vi "2ndOrderTF_v1.vi"(7 "Enable?":bool, 9 "Denominator":fxp<+/-,18,3>[](array[numeric])=[0.0, 0.0], 10 "Numerator":fxp<+/-,18,3>[](array[numeric])=[0.0, 0.0, 0.0], 11 "Input":fxp<+/-,25,4>) -> (3 "Output":fxp<+/-,25,4> format="%.29g")   [LabVIEW 2017, in "FPGA Controllers.lvlib"]
doc: "2nd order TF. Use this for implementing a notch filter.\n\nImplements, u(k) = a0*e(k-2) + a1*e(k-1) + a2*e(k) - b0*u(k-2) - b1*u(k-1)\n\nSet parameters, Num = a0, a1, a2 and Den = b0, b1"
uses:
  FPGA Controllers.lvlib
  <vilib>/rvi/FXPMathLib/basic elements/FxpDiscreteDelay/XNode/nifxpmath_DiscreteDelay.xnode
  <vilib>/Platform/TimedLoop/XDataNode/XDataNode.xnode
  <vilib>/Platform/TimedLoop/XDataNode/nitl_modes.ctl
  <vilib>/Platform/TimedLoop/XDataNode/XDNodeRunTimeDep.lvlib
  <vilib>/Platform/TimedLoop/XDataNode/wakeup.ctl
  <vilib>/Platform/TimedLoop/XDataNode/timing_clust.ctl
  <vilib>/rvi/FXPMathLib/FxpMul/XNode/nifxpmath_Multiplier.xnode
  <vilib>/rvi/FXPMathLib/sim/FxpSim.dll
  <vilib>/rvi/FXPMathLib/FxpAdd/XNode/nifxpmath_Add.xnode
  <vilib>/rvi/FXPMathLib/FxpSub/XNode/nifxpmath_Sub.xnode
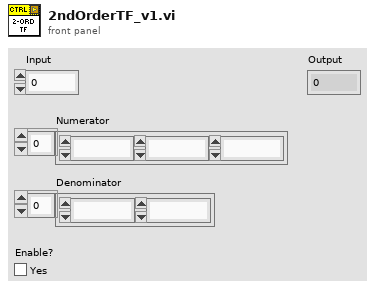
[diagram p1: front panel]
types:
  T1 = typedef "XDNodeRunTimeDep.lvlib/timing_clust.ctl" = cluster{"Expected End [f-1]":u64, "Actual End [f-1]":u64, "Finished Late? [f-1]":bool, "Expected End [i-1]":u64, "Actual End [i-1]":u64, "Finished Late? [i-1]":bool, "Expected Start [i]":u64, "Actual Start [i]":u64, "Expected Start [f]":u64, "Actual Start [f]":u64, "Source Name":string, "Structure Name":string, "Period":i64, "Deadline":i64, "Offset":i64, "Start":i64, "Priority":i32, "Timeout":i32, "Mode":T2, "Wakeup Reason":T3, "Error":errorcluster, "Source Type":string, "Secondary Source Type":string, "Global End Time":u64, "Global Start Time":u64, "Frame Duration":u64, "Iteration Duration":u64, "Assigned CPU":i32, "I/O Scan Engine Mode":u32}
  T2 = typedef "XDNodeRunTimeDep.lvlib/nitl_modes.ctl" = enum32{"No Change", "Process missed periods, maintain original phase", "Discard missed periods, maintain original phase", "Process missed periods, ignore original phase", "Discard missed periods, ignore original phase"}
  T3 = typedef "XDNodeRunTimeDep.lvlib/wakeup.ctl" = enum32{"Normal", "Aborted", "Asynchronous wakeup", "Timing source error", "Timed loop error", "Timeout"}
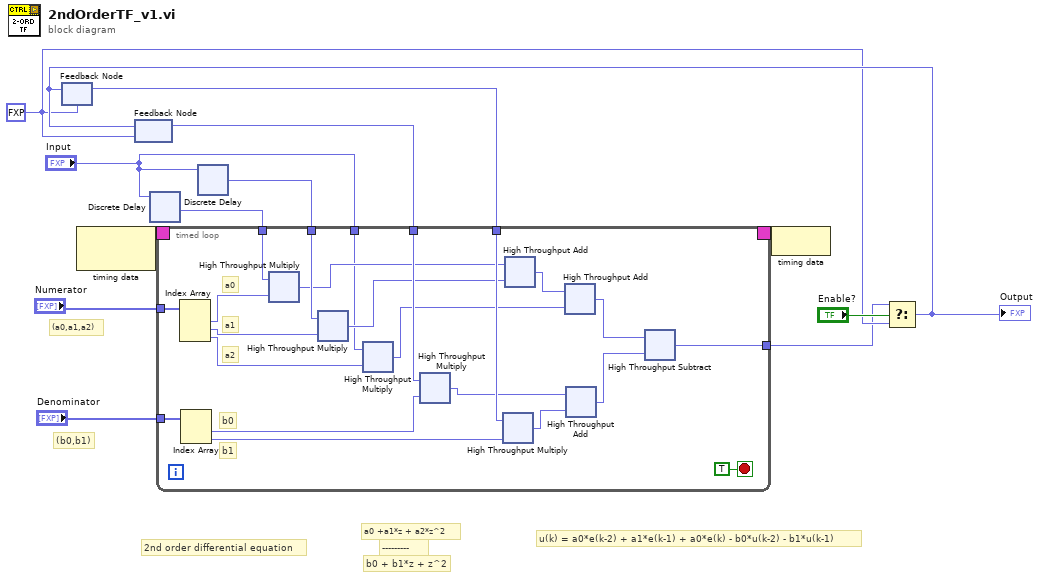
[diagram p0: block diagram]
diagram:
  w4 = fxp<+/-,25,4> 0.0 ("Input")
  # "2nd order differential equation"
  # "u(k) = a0*e(k-2) + a1*e(k-1) + a0*e(k) - b0*u(k-2) - b1*u(k-1)"
  # "(b0,b1)"
  # "(a0,a1,a2)"
  # "b0 + b1*z + z^2"
  # "a0 +a1*z + a2*z^2"
  # "---------"
  n1 = feedback #1(w4) -> (w5:fxp<+/-,25,4>)
  n2 = node-c288() -> (w11:T1)  [unwired: 1 in]
  n3 = feedback #2(w4) -> (w6:fxp<+/-,25,4>)
  n4 = xnode ("Discrete Delay")("D"="Input") -> ("Q"=w7:fxp<+/-,25,4>)
  n5 = xnode ("Discrete Delay")("D"="Input") -> ("Q"=w2:fxp<+/-,25,4>)
  n6 = timed-loop {
    timing: w11 -> [_]
    timing-out: [_] -> w10
    tunnel: "Numerator" -> [w34]
    tunnel: "Denominator" -> [w33]
    tunnel: w2 -> [w30]
    tunnel: w7 -> [w29]
    tunnel: w6 -> [w26]
    tunnel: w5 -> [w25]
    tunnel: [w20] -> w3
    tunnel: "Input" -> [w18]
    stop <- TRUE stop-if-true
    # "a2"
    # "b0"
    # "b1"
    # "a1"
    # "a0"
    n7 = Index Array(array=w34) -> (element #1=w32:fxp<+/-,18,3>, element #2=w31:fxp<+/-,18,3>, element #3=w17:fxp<+/-,18,3>)  [unwired: 3 in]
    n8 = Index Array(array=w33) -> (element #1=w27:fxp<+/-,18,3>, element #2=w28:fxp<+/-,18,3>)  [unwired: 2 in]
    n9 = xnode ("High Throughput Multiply")("x"=w29, "y"=w32) -> ("x*y"=w24:fxp<+/-,43,7>)
    n10 = xnode ("High Throughput Multiply")("x"=w30, "y"=w31) -> ("x*y"=w19:fxp<+/-,43,7>)
    n11 = xnode ("High Throughput Multiply")("x"=w18, "y"=w17) -> ("x*y"=w16:fxp<+/-,43,7>)
    n12 = xnode ("High Throughput Multiply")("x"=w26, "y"=w27) -> ("x*y"=w23:fxp<+/-,43,7>)
    n13 = xnode ("High Throughput Multiply")("x"=w25, "y"=w28) -> ("x*y"=w22:fxp<+/-,43,7>)
    n14 = xnode ("High Throughput Add")("x"=w24, "y"=w19) -> ("x+y"=w15:fxp<+/-,44,8>)
    n15 = xnode ("High Throughput Add")("x"=w15, "y"=w16) -> ("x+y"=w14:fxp<+/-,45,9>)
    n16 = xnode ("High Throughput Add")("x"=w23, "y"=w22) -> ("x+y"=w21:fxp<+/-,44,8>)
    n17 = xnode "High Throughput Subtract"("x"=w14, "y"=w21) -> ("x-y"=w20:fxp<+/-,25,4>)
  }
  n18 = node-c288(w10) -> ()
  n19 = Select(t=w3, s="Enable?", f=w4) -> (s? t:f=w12:fxp<+/-,25,4>)
  "Output" <- w12
  n20 = feedback-in #1(w12) -> ()
  n21 = feedback-in #2(w12) -> ()
